vi "Read Update once lower.vi"(8 "error in (no error)":errorcluster, 11 "Scope5761":refnum<class "Scope5782_six_channel.lvclass">) -> (0 "error out":errorcluster, 2 "Update once lower":bool, 3 "Scope5761":refnum<class "Scope5782_six_channel.lvclass">)   [LabVIEW 2018, in "Scope5782_six_channel.lvclass"]
uses:
  Scope5782_six_channel.lvclass
  Scope5782_six_channel.lvclass/Scope5782_six_channel.ctl
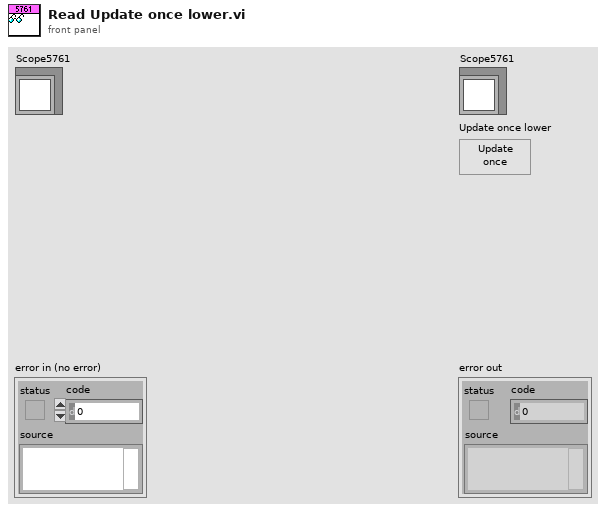
[diagram p1: front panel]
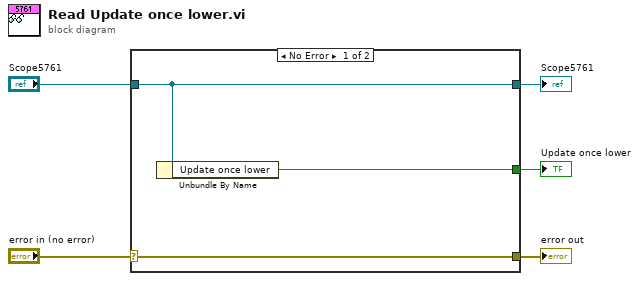
[diagram p0: block diagram]
diagram:
  n1 = case shown="No Error" "error in (no error)" {
    selector: "error in (no error)" -> [w8 w9]
    tunnel: [w8 w9] -> w4
    tunnel: [w7 w10] -> w2
    tunnel: "Scope5761" -> [w7 w10]
    tunnel: [w6 _] -> w1
    frame No Error {
      n2 = Unbundle By Name(w7) -> ("Update once lower"=w6:bool)
    }
    frame Error {
    }
  }
  "error out" <- w4
  "Scope5761" <- w2
  "Update once lower" <- w1
